vi "mainActivity_glb.vi"() -> ()   [LabVIEW 2014]
panel:
  in  "侧边栏显示信息_mainActivity":string[][](array[string])
  in  "stop":bool
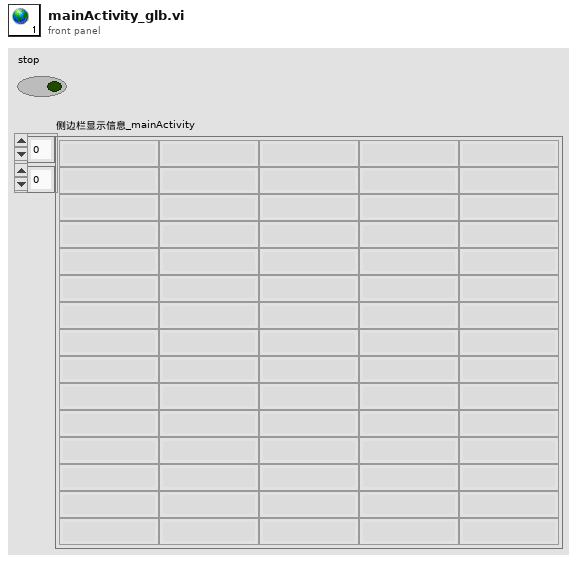
[diagram p1: front panel]
diagram:
